vi "3D potential flow (non-lifting bodies), top level.vi"(0 "STL geometry file path":path=path "C:/EnFlo Software/Anemometry/Utilities/Probe blockage potential flow sim/test stl files/Ring torus.stl", 1 "U_inf":sgl[](array[numeric])=[1.0, 0.0, 0.0], 2 "solver method":u8(ring)=1 items=["Jacobi (rel.)", "Jacobi (abs.)", "Gauss-Seidel (rel.)", "Gauss-Seidel (abs.)", "NI solver"], 3 "res. tol.":dbl=0.01 format="%#_6e", 4 "max. iters":i32=1000, 5 "P_meas":sgl[](array[numeric])=[0.0, 0.0, 0.0], 6 "P_start":sgl[](array[numeric])=[0.0, -10.0, 0.0], 7 "P_end":sgl[](array[numeric])=[0.0, 10.0, 0.0], 8 "Virtual particle trace":bool=TRUE, 9 "N_pts":i32=100, 10 "Virtual traverse profile":bool=TRUE, 11 "Coordinate to plot":u8(ring)=1 items=["x", "y", "z"], 12 "Get velocity at P_meas":bool=TRUE, 13 "P_start (trace)":sgl[](array[numeric])=[0.0, 0.0, 0.0], 14 "Get surface Cp":bool=TRUE, 15 "dt":sgl=0.01, 16 "Load geometry and solve":bool=TRUE, 17 "r_max":sgl=10.0) -> (20 "Velocity at P_meas":sgl[](array[numeric]), 22 "Virtual traverse profile out":T4, 24 "Particle trace out":T3, 26 "Panel ctrl pts.":sgl[][](array[numeric]), 27 "Cp":sgl[](array[numeric]))   [LabVIEW 2017]
uses:
  <vilib>/Utility/miscctls.llb/LV3DPointTypeDef.ctl
  ctls/Triangle panel.ctl
  <vilib>/Utility/miscctls.llb/LVRGBAColorTypeDef.ctl
panel:
  out "3D Picture":refnum<vi>(3d-picture)
  out "Cp(x, y, z)":cluster{"Panel ctrl pts.":sgl[], "Cp":sgl[]}[](graph)
  in  "Render to full-screen":bool
  out "Pcols":T1[](array[typedef])
  out "Ls2":sgl[][](array[numeric])
  out "Ls1":sgl[][](array[numeric])
  out "Panel triangles out":T2[](array[typedef])
  in  "Up direction":T5={"X"=0.0, "Y"=0.0, "Z"=1.0}
  in  "Camera target":T5={"X"=3.0, "Y"=0.0, "Z"=0.0}
  in  "Camera position":T5={"X"=-5.0, "Y"=5.0, "Z"=5.0}
  in  "Cp_max clamp (for 3D rendering only)":sgl=1.0 format="%#_6f"
  in  "Cp_min clamp (for 3D rendering only)":sgl=-4.0 format="%#_6f"
  in  "Render mode":T6(ring)=enum."Polygons"
  out "Cp_max":sgl
  out "Cp_min":sgl
  out "sys. residual":sgl
  out "Particle trace":cluster{sgl[], sgl[]}[](graph)
  out "N panels":i32
  out "Virtual traverse profile":cluster{sgl[], sgl[]}[](graph)
  out "Converged?":bool
  out "Iterations":i32
  # "U"
  # "V"
  # "W"
  # "x"
  # "U"
  # "y"
  # "V"
  # "z"
  # "W"
  # "Written by Paul Nathan, 26/10/2017"
  # "Vertices"
  # "Edges"
  # "Unit normal"
  # "Control point"
  # "Edge\nlinks \n(tri index)"
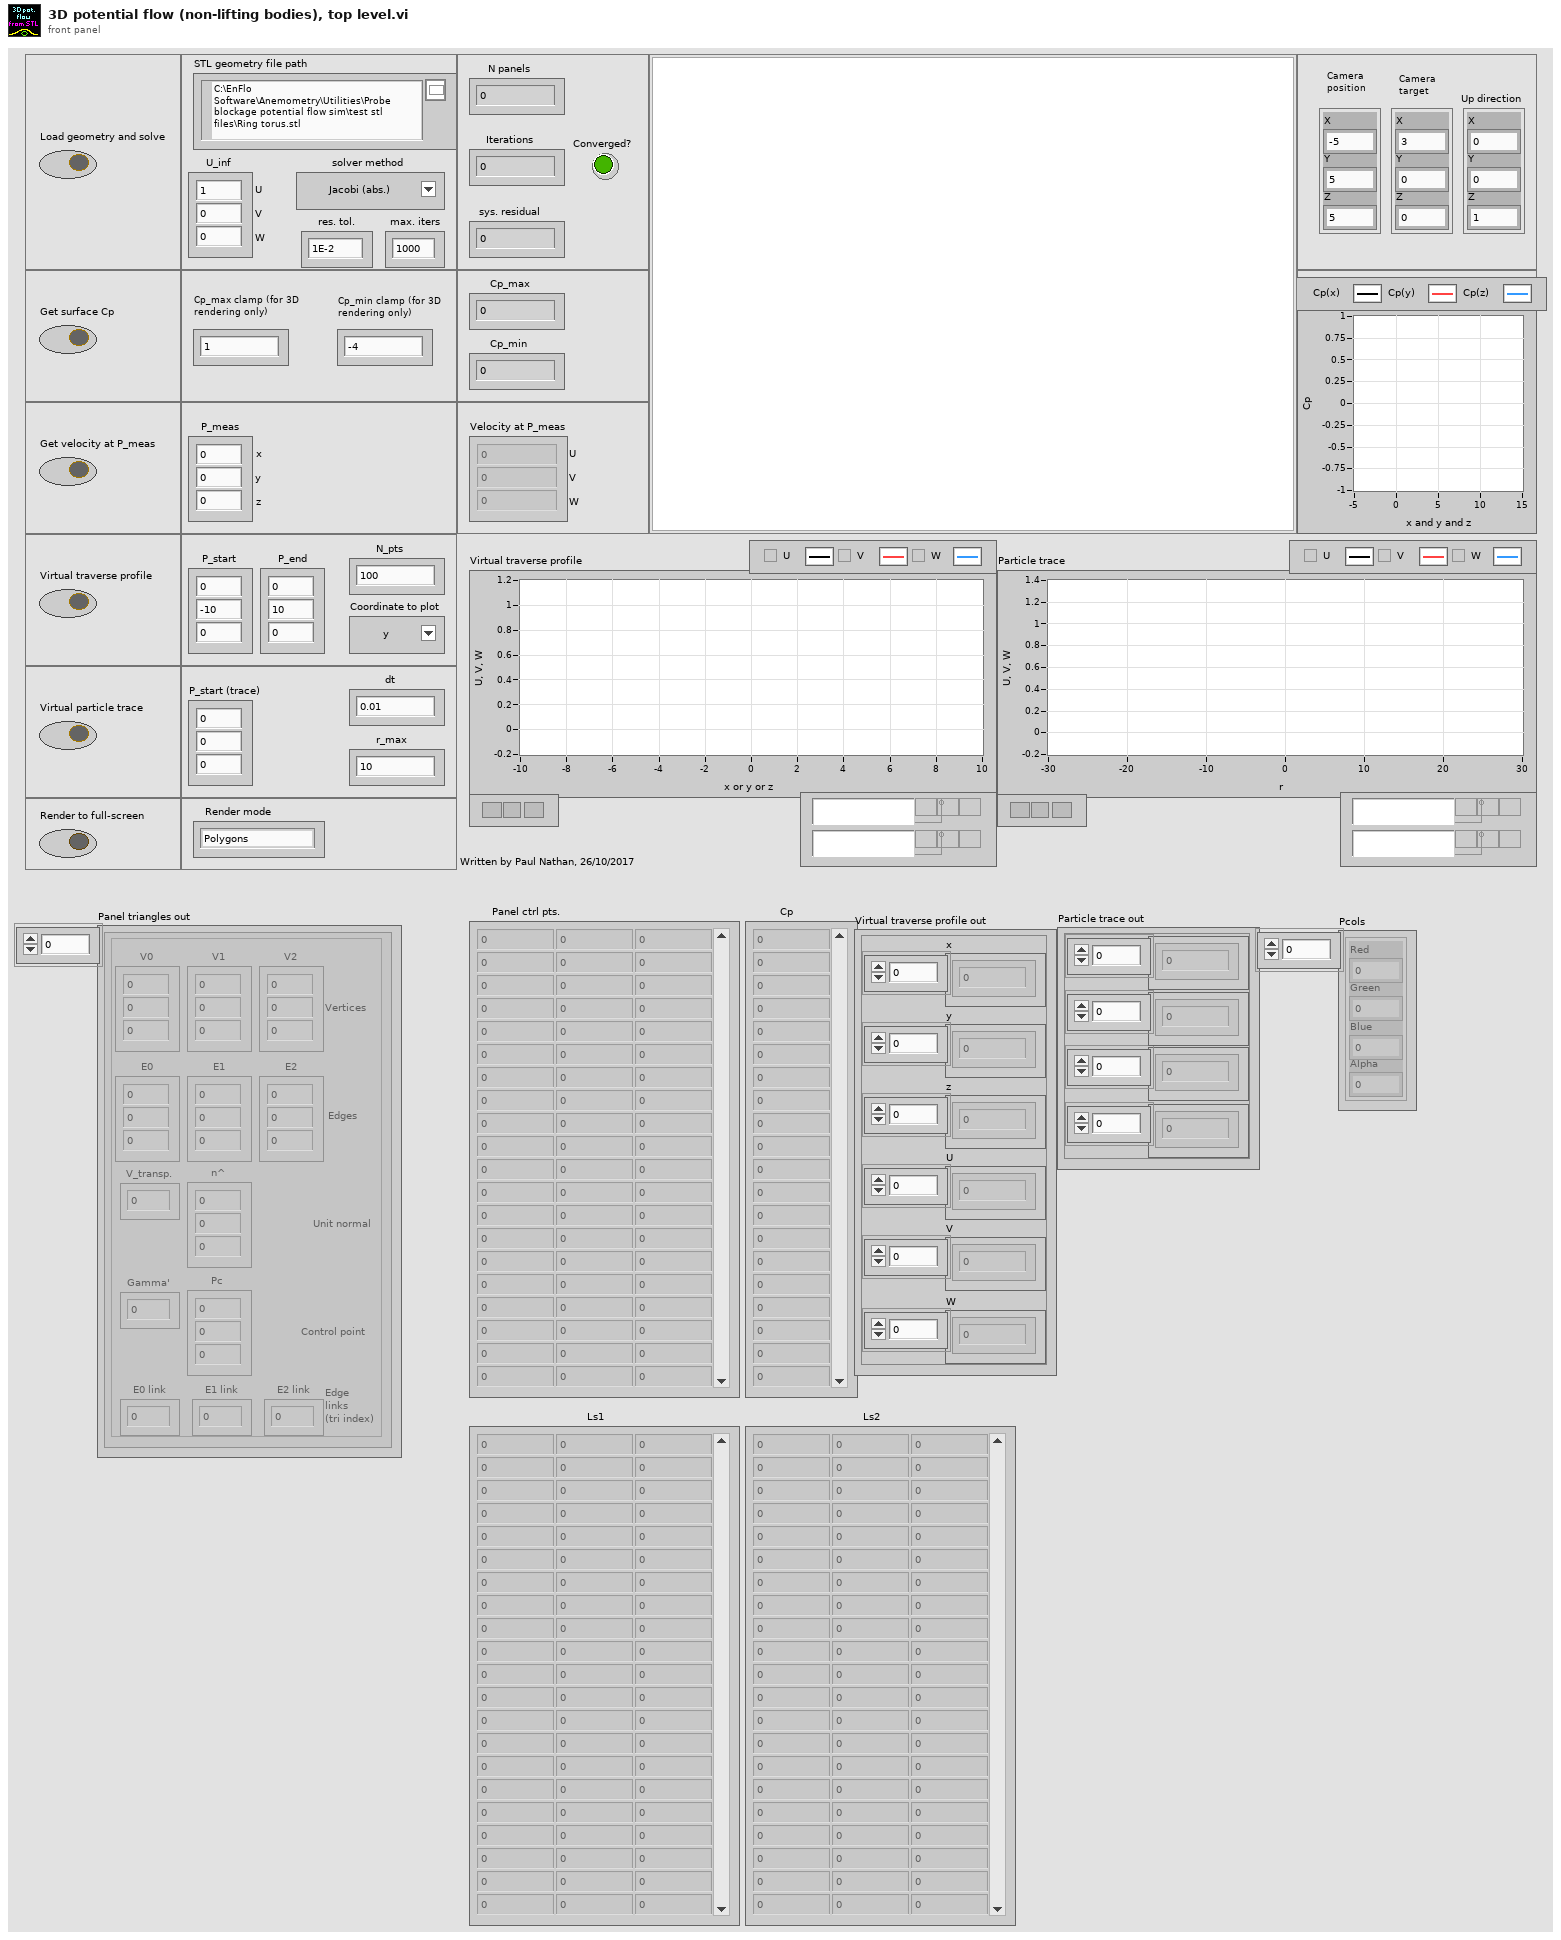
[diagram p1: front panel]
types:
  T1 = typedef "LVRGBAColorTypeDef.ctl" = cluster{"Red":sgl, "Green":sgl, "Blue":sgl, "Alpha":sgl}
  T2 = typedef "Triangle panel.ctl" = cluster{"V0":sgl[], "V1":sgl[], "V2":sgl[], "E0":sgl[], "E1":sgl[], "E2":sgl[], "n^":sgl[], "Pc":sgl[], "Gamma'":sgl, "V_transp.":sgl, "E0 link":i32, "E1 link":i32, "E2 link":i32}
  T3 = cluster{"Array":sgl[], "Array":sgl[], "Array":sgl[], "Array":sgl[]}
  T4 = cluster{"x":sgl[], "y":sgl[], "z":sgl[], "U":sgl[], "V":sgl[], "W":sgl[]}
  T5 = typedef "LV3DPointTypeDef.ctl" = cluster{"X":sgl, "Y":sgl, "Z":sgl}
  T6 = enum16{"Inherit Value", "Points", "Wireframe", "Polygons"}
  T7 = enum16{"None", "Spherical", "Flying", "Oriented"}
  T8 = typedef "LVRectTypeDef.ctl" = cluster{"Left":i16, "Top":i16, "Right":i16, "Bottom":i16}
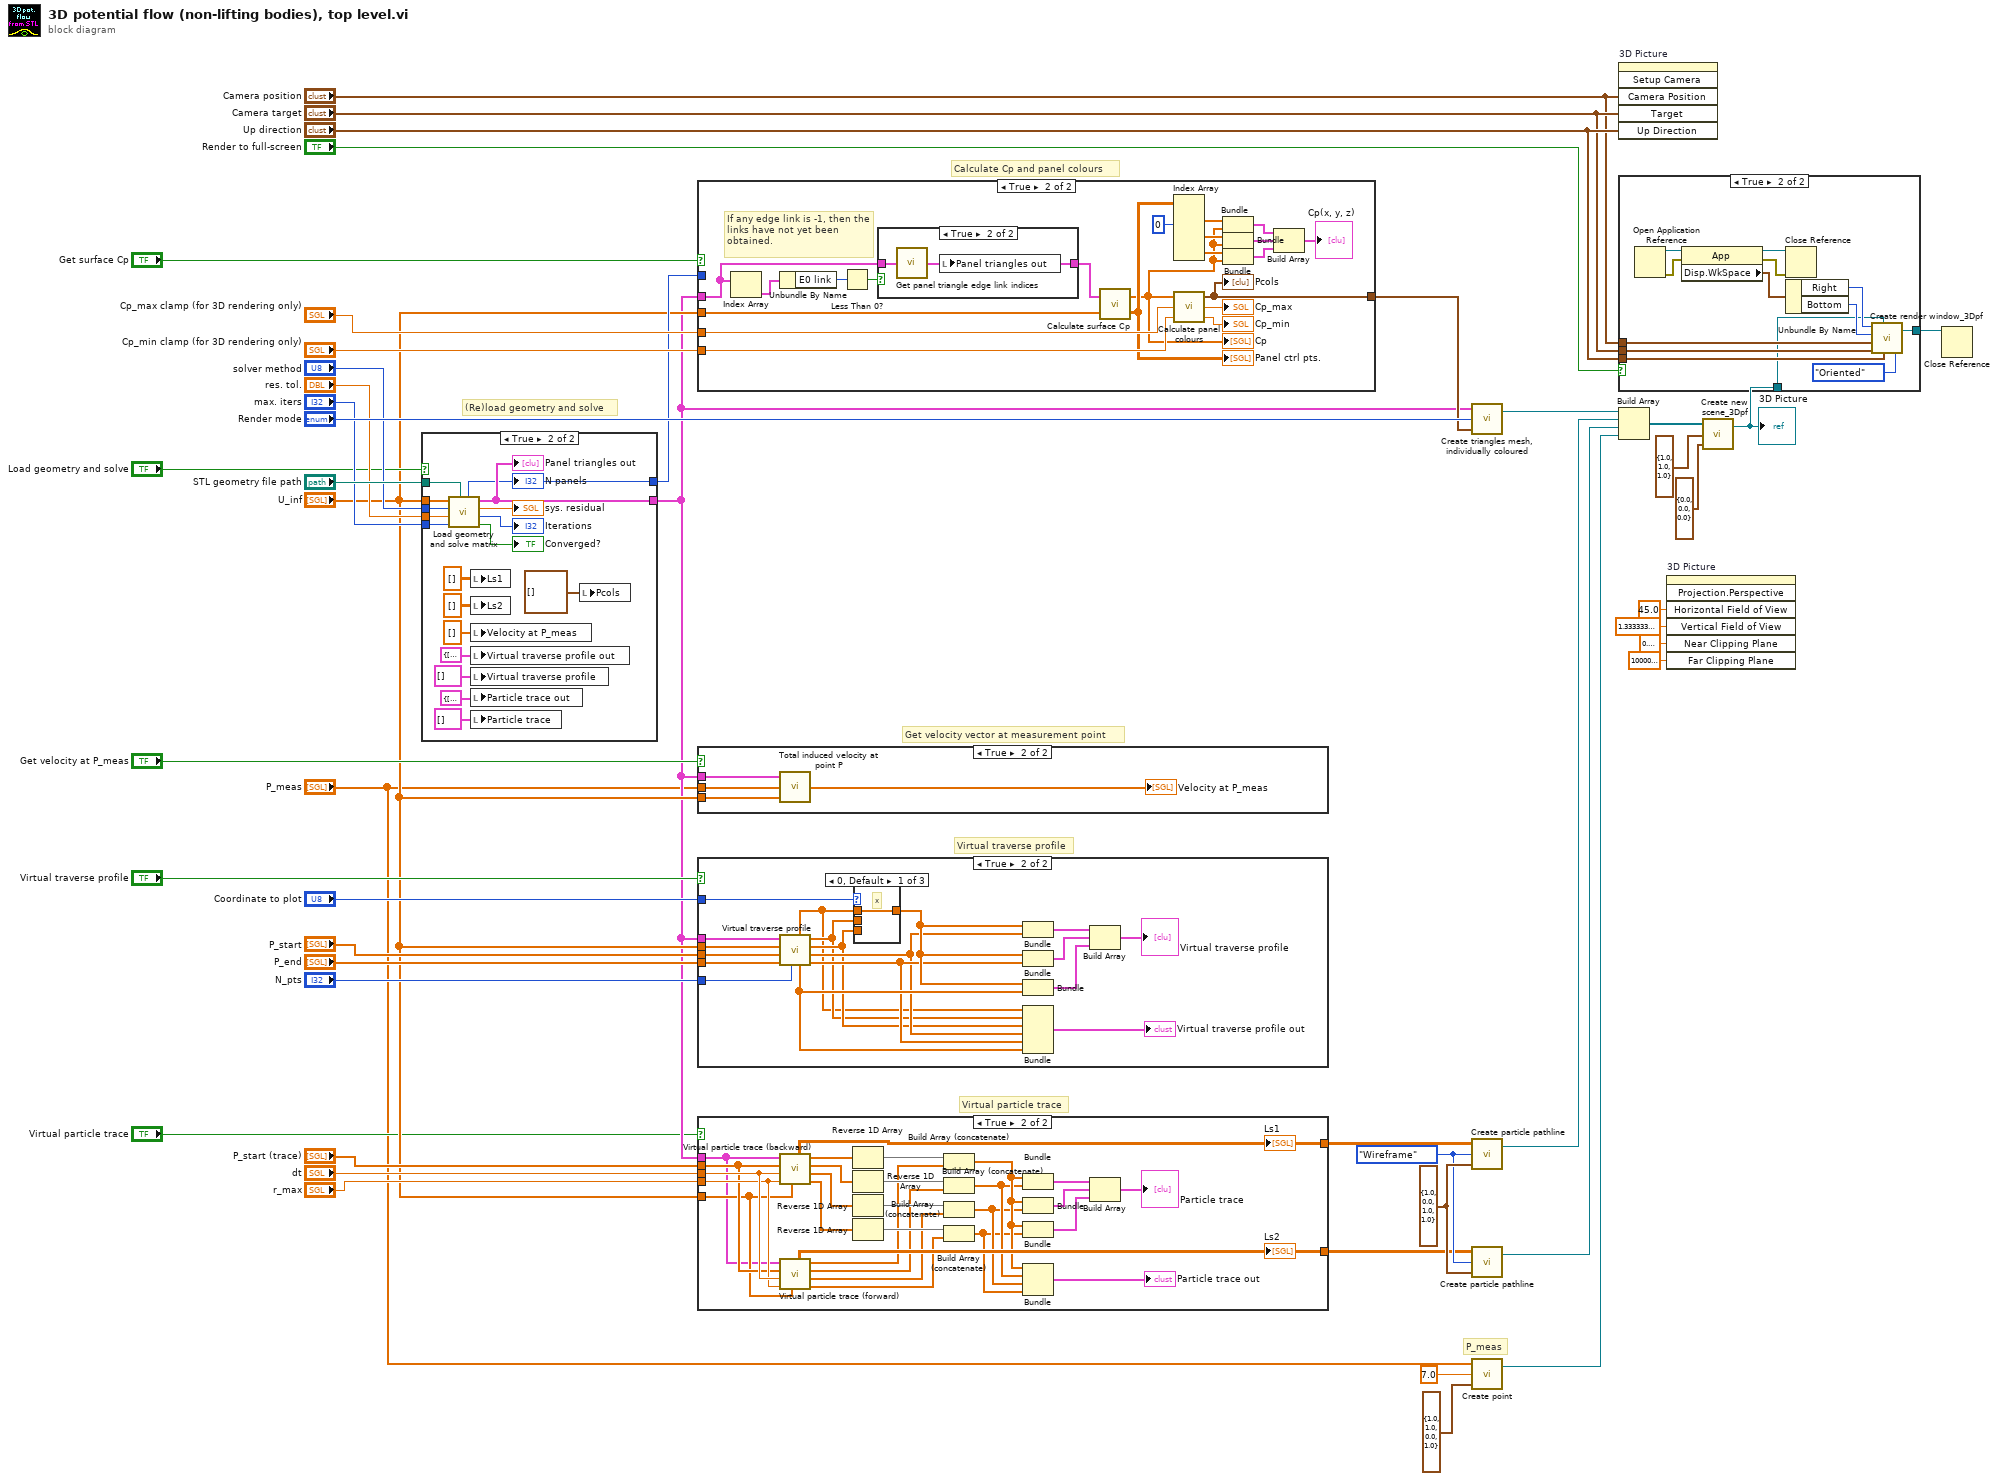
[diagram p0: block diagram]
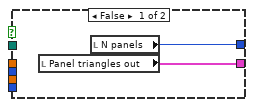
[diagram p3: hidden frame]
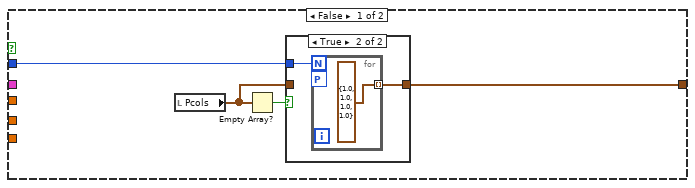
[diagram p4: hidden frame]
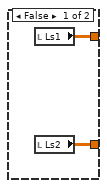
[diagram p7: hidden frame]
diagram:
  w12 = T1 {"Red"=1.0, "Green"=0.0, "Blue"=1.0, "Alpha"=1.0} ("Colour")
  w11 = T6."Wireframe" ("Render mode")
  # "(Re)load geometry and solve"
  # "Get velocity vector at measurement point"
  # "Calculate Cp and panel colours"
  # "Virtual traverse profile"
  # "P_meas"
  # "Virtual particle trace"
  n1 = case shown="True" "Load geometry and solve" {
    tunnel: "STL geometry file path" -> [_ w67]
    tunnel: "solver method" -> [_ w66]
    tunnel: "res. tol." -> [_ w65]
    tunnel: "max. iters" -> [_ w64]
    tunnel: [w48 w60] -> w13
    tunnel: "U_inf" -> [_ w59]
    tunnel: [w49 w58] -> w18
    frame False {
      n2 = local read "Panel triangles out"() -> (w48:T2[])
      n3 = local read "N panels"() -> (w49:i32)
    }
    frame True {
      n4 = call "Load geometry and solve matrix.vi"("STL geometry file path"=w67, "max. iters"=w64, "res. tol."=w65, "solver method"=w66, "U_inf"=w59) -> ("Converged?"=→"Converged?":bool, "Iterations"=→"Iterations":i32, "sys. residual"=→"sys. residual":sgl, "Panel triangles out"=w60:T2[], "N panels"=w58:i32)  [unwired: 1 in, 1 out]
      "N panels" <- w58
      "Panel triangles out" <- w60
      n5 = local write "Ls1"(sgl[][] [] ("Ls1")) -> ()
      n6 = local write "Ls2"(sgl[][] [] ("Ls2")) -> ()
      n7 = local write "Velocity at P_meas"(sgl[] [] ("(U, V, W) at P_meas")) -> ()
      n8 = local write "Virtual traverse profile out"(T4 {"x"=[], "y"=[], "z"=[], "U"=[], "V"=[], "W"=[]} ("Virtual traverse profile out")) -> ()
      n9 = local write "Virtual traverse profile"(cluster{sgl[], sgl[]}[] [] ("Virtual traverse profile")) -> ()
      n10 = local write "Particle trace out"(T3 {"Array"=[], "Array"=[], "Array"=[], "Array"=[]} ("Particle trace out")) -> ()
      n11 = local write "Particle trace"(cluster{sgl[], sgl[]}[] [] ("Particle trace")) -> ()
      n12 = local write "Pcols"(T1[] [] ("Pcols")) -> ()
    }
  }
  n13 = case shown="True" "Get surface Cp" {
    tunnel: "Cp_max clamp (for 3D rendering only)" -> [_ w96]
    tunnel: "Cp_min clamp (for 3D rendering only)" -> [_ w95]
    tunnel: [w71 w94] -> w31
    tunnel: w13 -> [_ w87]
    tunnel: "U_inf" -> [_ w91]
    tunnel: w18 -> [w70 _]
    frame False {
      n14 = local read "Pcols"() -> (w68:T1[])
      n15 = Empty Array?(array=w68) -> (empty?=w69:bool)
      n16 = case shown="True" w69 {
        tunnel: [w72 w74] -> w71
        tunnel: w70 -> [_ w73]
        tunnel: w68 -> [w72 _]
        frame False {
        }
        frame True {
          n17 = for {
            N: w73 -> [_]
            tunnel: [T1 {"Red"=1.0, "Green"=1.0, "Blue"=1.0, "Alpha"=1.0} ("Colour out")] -> w74 mode=indexing
            workers-P: _ -> [_]
          }
        }
      }
    }
    frame True {
      # "If any edge link is -1, then the links have not yet been obtained."
      n18 = Index Array(array=w87) -> (element=w88:T2)  [unwired: 1 in]
      n19 = Unbundle By Name(w88) -> ("E0 link"=w89:i32)
      n20 = Less Than 0?(x=w89) -> (x < 0?=w90:bool)
      n21 = case shown="True" w90 {
        tunnel: [w97 w98] -> w86
        tunnel: w87 -> [w97 w99]
        frame False {
        }
        frame True {
          n22 = call "Get panel triangle edge link indices.vi"("Panel triangles in"=w99) -> ("Panel triangles out"=w98:T2[])
          n23 = local write "Panel triangles out"(w98) -> ()
        }
      }
      n24 = call "Calculate surface Cp.vi"("U_inf"=w91, "Panel triangles in"=w86) -> ("Panel ctrl pts."=w77:sgl[][], "Cp"=w76:sgl[])
      "Panel ctrl pts." <- w77
      "Cp" <- w76
      n25 = Index Array(array=w77, index (col) #1=0 ("disabled index (col)")) -> (element #1=w79:sgl[], element #2=w80:sgl[], element #3=w81:sgl[])  [unwired: 5 in]
      n26 = call "Calculate panel colours.vi"("Cp_min clamp (for 3D rendering)"=w95, "Cp_max clamp (for 3D rendering)"=w96, "Cp"=w76) -> ("Cp_min"=→"Cp_min":sgl, "Cp_max"=→"Cp_max":sgl, "Panel colours"=w94:T1[])
      "Pcols" <- w94
      n27 = Bundle("Panel ctrl pts."=w79, "Cp"=w76) -> (w82:cluster{"Panel ctrl pts.":sgl[], "Cp":sgl[]})  [unwired: 1 in]
      n28 = Bundle("Panel ctrl pts."=w80, "Cp"=w76) -> (w83:cluster{"Panel ctrl pts.":sgl[], "Cp":sgl[]})  [unwired: 1 in]
      n29 = Bundle("Panel ctrl pts."=w81, "Cp"=w76) -> (w84:cluster{"Panel ctrl pts.":sgl[], "Cp":sgl[]})  [unwired: 1 in]
      n30 = Build Array(w82, w83, w84) -> (→"Cp(x, y, z)":cluster{"Panel ctrl pts.":sgl[], "Cp":sgl[]}[])
    }
  }
  n31 = case shown="True" "Get velocity at P_meas" {
    tunnel: "P_meas" -> [_ w103]
    tunnel: w13 -> [_ w102]
    tunnel: "U_inf" -> [_ w101]
    frame False {
    }
    frame True {
      n32 = call "Total induced velocity at point P.vi"("U_inf"=w101, "P"=w103, "Triangle panels"=w102) -> ("(U, V, W) at P"=→"Velocity at P_meas":sgl[])
    }
  }
  n33 = case shown="True" "Virtual traverse profile" {
    tunnel: "N_pts" -> [_ w118]
    tunnel: "P_end" -> [_ w117]
    tunnel: "Coordinate to plot" -> [_ w116]
    tunnel: w13 -> [_ w115]
    tunnel: "P_start" -> [_ w114]
    tunnel: "U_inf" -> [_ w113]
    frame False {
    }
    frame True {
      n34 = call "Virtual traverse profile.vi"("N_pts"=w118, "P_end"=w117, "P_start"=w114, "U_inf"=w113, "Panel triangles in"=w115) -> ("V"=w109:sgl[], "U"=w108:sgl[], "z"=w107:sgl[], "y"=w106:sgl[], "W"=w110:sgl[], "x"=w105:sgl[])  [unwired: 1 in]
      n35 = case shown="0, Default" w116 {
        tunnel: [w122 w123 w124] -> w111
        tunnel: w105 -> [w122 _ _]
        tunnel: w106 -> [_ w123 _]
        tunnel: w107 -> [_ _ w124]
        frame 0, Default {
          # "x"
        }
        frame 1 {
          # "y"
        }
        frame 2 {
          # "z"
        }
      }
      n36 = Bundle("z"=w111, "U"=w108) -> (w121:cluster{"z":sgl[], "U":sgl[]})  [unwired: 1 in]
      n37 = Bundle("z"=w111, "V"=w109) -> (w120:cluster{"z":sgl[], "V":sgl[]})  [unwired: 1 in]
      n38 = Bundle("z"=w111, "W"=w110) -> (w119:cluster{"z":sgl[], "W":sgl[]})  [unwired: 1 in]
      n39 = Bundle("x"=w105, "y"=w106, "z"=w107, "U"=w108, "V"=w109, "W"=w110) -> (→"Virtual traverse profile out":T4)  [unwired: 1 in]
      n40 = Build Array(w121, w120, w119) -> (→"Virtual traverse profile":cluster{"z":sgl[], "W":sgl[]}[])
    }
  }
  n41 = case shown="True" "Virtual particle trace" {
    tunnel: "dt" -> [_ w154]
    tunnel: "r_max" -> [_ w153]
    tunnel: "P_start (trace)" -> [_ w152]
    tunnel: "U_inf" -> [_ w151]
    tunnel: w13 -> [_ w150]
    tunnel: [w125 w149] -> w10
    tunnel: [w126 w148] -> w9
    frame False {
      n42 = local read "Ls1"() -> (w126:sgl[][])
      n43 = local read "Ls2"() -> (w125:sgl[][])
    }
    frame True {
      n44 = call "Virtual particle trace (backward).vi"("U_inf"=w151, "r_max"=w153, "dt"=w154, "P_start"=w152, "Panel triangles in"=w150) -> ("W"=w140:sgl[], "V"=w141:sgl[], "U"=w142:sgl[], "r"=w143:sgl[], "Points"=w148:sgl[][])  [unwired: 1 in, 1 out]
      "Ls1" <- w148
      n45 = call "Virtual particle trace (forward).vi"("U_inf"=w151, "r_max"=w153, "dt"=w154, "P_start"=w152, "Panel triangles in"=w150) -> ("W"=w132:sgl[], "V"=w133:sgl[], "U"=w134:sgl[], "r"=w135:sgl[], "Points"=w149:sgl[][])  [unwired: 1 in, 1 out]
      "Ls2" <- w149
      n46 = Reverse 1D Array(array=w143) -> (reversed array=w139:sgl[])
      n47 = Reverse 1D Array(array=w142) -> (reversed array=w138:sgl[])
      n48 = Reverse 1D Array(array=w141) -> (reversed array=w137:sgl[])
      n49 = Reverse 1D Array(array=w140) -> (reversed array=w136:sgl[])
      n50 = Build Array (concatenate)(w139, w135) -> (w131:sgl[])
      n51 = Build Array (concatenate)(w138, w134) -> (w130:sgl[])
      n52 = Build Array (concatenate)(w137, w133) -> (w129:sgl[])
      n53 = Build Array (concatenate)(w136, w132) -> (w128:sgl[])
      n54 = Bundle(w131, w130) -> (w144:cluster{sgl[], sgl[]})  [unwired: 1 in]
      n55 = Bundle(w131, w129) -> (w146:cluster{sgl[], sgl[]})  [unwired: 1 in]
      n56 = Bundle(w131, w128) -> (w147:cluster{sgl[], sgl[]})  [unwired: 1 in]
      n57 = Bundle(w131, w130, w129, w128) -> (→"Particle trace out":cluster{sgl[], sgl[], sgl[], sgl[]})  [unwired: 1 in]
      n58 = Build Array(w144, w146, w147) -> (→"Particle trace":cluster{sgl[], sgl[]}[])
    }
  }
  n59 = call "Create triangles mesh, individually coloured.vi"("Colours array"=w31, "Render mode"="Render mode", "Triangles array"=w13) -> ("Triangle mesh out"=w35:refnum<vi>)  [unwired: 1 out]
  n60 = call "Create particle pathline.vi"("Colour"=w12, "Render mode"=w11, "Points"=w9) -> ("Pathline out"=w44:refnum<vi>)  [unwired: 1 out]
  n61 = call "Create particle pathline.vi"("Colour"=w12, "Render mode"=w11, "Points"=w10) -> ("Pathline out"=w43:refnum<vi>)  [unwired: 1 out]
  n62 = call "Create point.vi"("Colour"=T1 {"Red"=1.0, "Green"=1.0, "Blue"=0.0, "Alpha"=1.0}, "Point size"=7.0, "Point"="P_meas") -> ("Point out"=w40:refnum<vi>)  [unwired: 1 out]
  n63 = invoke on="3D Picture" class="SceneGraphDisp (strict)" method="Setup Camera"("Camera Position"="Camera position", "Target"="Camera target", "Up Direction"="Up direction") -> ()  [unwired: 3 in, 6 out]
  n64 = Build Array(w35, w44, w43, w40) -> (w34:refnum<vi>[])
  n65 = invoke on="3D Picture" class="SceneGraphDisp (strict)" method="Projection.Perspective"("Horizontal Field of View"=sgl 45.0 ("Field of View"), "Vertical Field of View"=sgl 1.3333334 ("Aspect Ratio"), "Near Clipping Plane"=sgl 0.1, "Far Clipping Plane"=sgl 1000000.0) -> ()  [unwired: 3 in, 7 out]
  n66 = call "Create new scene_3Dpf.vi"("Translation"=cluster{"X":sgl, "Y":sgl, "Z":sgl} {"X"=0.0, "Y"=0.0, "Z"=0.0}, "Scale"=cluster{"X":sgl, "Y":sgl, "Z":sgl} {"X"=1.0, "Y"=1.0, "Z"=1.0}, "Scene objects array"=w34) -> ("Scene out"=w3:refnum<vi>)  [unwired: 1 out]
  "3D Picture" <- w3
  n67 = case shown="True" "Render to full-screen" {
    tunnel: "Camera position" -> [_ w168]
    tunnel: "Camera target" -> [_ w167]
    tunnel: "Up direction" -> [_ w166]
    tunnel: w3 -> [w155 w157]
    tunnel: [w155 w156] -> w2
    frame False {
    }
    frame True {
      n68 = Open Application Reference() -> (0:w162:errorcluster, 3:w161:refnum<vi>)  [unwired: 4 in]
      n69 = property class="App"(reference=w161, error in=w162) -> (reference out=w163:refnum<vi>, error out=w164:errorcluster, "Disp.WkSpace"=w165:T8)
      n70 = Close Reference(reference=w163, error in (no error)=w164) -> ()  [unwired: 1 out]
      n71 = Unbundle By Name(w165) -> ("Right"=w159:i16, "Bottom"=w160:i16)
      n72 = call "Create render window_3Dpf.vi"("Camera Controller:Type"=T7."Oriented", "Up Direction"=w166, "Scene in"=w157, "Target"=w167, "Camera Position"=w168, "Height"=w160, "Width"=w159) -> ("Scene out"=w156:refnum<vi>)
    }
  }
  n73 = Close Reference(reference=w2) -> ()  [unwired: 1 in, 1 out]
